vi "UTILITY Delay mS.vi"(11 "Error In":errorcluster, 13 "milliseconds to wait":u32) -> (15 "Error Out":errorcluster)   [LabVIEW 2018]
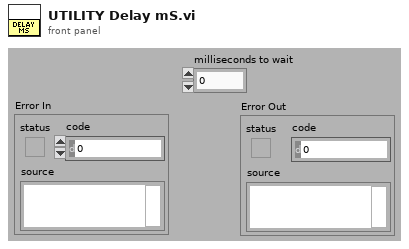
[diagram p1: front panel]
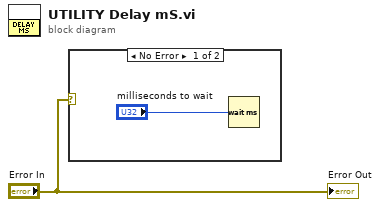
[diagram p0: block diagram]
diagram:
  n1 = case shown="No Error" "Error In" {
    frame No Error {
      n2 = Wait (ms)(milliseconds to wait="milliseconds to wait") -> ()  [unwired: 1 out]
    }
    frame Error {
    }
  }
  "Error Out" <- "Error In"
